vi "AB_Engine_Get_User_Build_Data.vi"(11 "Build in":refnum<class "AB_Build.lvclass">) -> (0 "Build Spec Name":string, 1 "Project Path":path, 2 "Main Destination":path, 3 "Build out":refnum<class "AB_Build.lvclass">, 4 "Target Name":string, 6 "Always Included VIs":path[](array[path]))   [LabVIEW 2020]
uses:
  <vilib>/AppBuilder/AB_Classes/Build/AB_Build.lvclass
  <vilib>/AppBuilder/AB_Classes/Source/AB_Source.lvclass
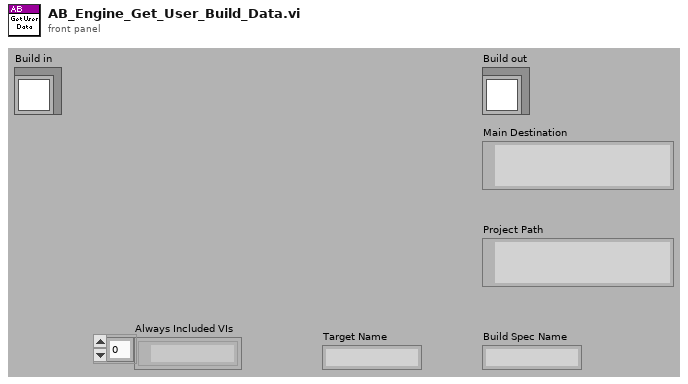
[diagram p1: front panel]
types:
  T1 = typedef "AB_Build.ctl" = cluster{"buildSpecName":string, "buildSpecDescription":string, "destinations":refnum<class "AB_Destination.lvclass">[], "exclusionOption":T2, "defaultLanguage":string, "supportedLanguages":string[], "excludedDirectories":path[], "buildContext":refnum<vi>, "buildObject":T3, "preview":bool, "programatic":bool, "progressBarEvents":T4, "userLog_Path":path, "preActionID":string, "preAction_Path":path, "postActionID":string, "postAction_Path":path, "eng_checkForBrokenVIs?":bool, "eng_verboseLinkerErrors?":bool, "localDest_Path":path, "targetDest_Path":path, "removeVIObject":u16, "cache":refnum<class "PreviewCache.lvclass">, "use cache":bool, "previewCache_ID":string, "buildCache_ID":string, "eng_TempLocalDest_Path":path, "eng_collectDependencies?":bool, "versionInfo":cluster{"buildVersion":cluster{"major":u16, "minor":u16, "patch":u16, "build":u16}, "autoIncrement":bool}, "eng_enableVIChecksums":bool}
  T2 = typedef "AB_Exclusion_Option.ctl" = cluster{"typedefs":bool, "polymorphicVIs":bool, "unusedLibraryItems":bool, "modifyLibraryFile":bool, "edit-timeDependencies":bool, "inlineVIs":bool, "dependent PPLs":bool, "dependent DLLs":bool}
  T3 = typedef "ItemRef.ctl" = u64
  T4 = typedef "provcom_ProgressBar_Events.ctl" = cluster{"newJob":refnum<user-event>, "newItem":refnum<user-event>, "errorMsg":T5, "cancel":refnum<user-event>}
  T5 = typedef "mxLvBuildError.ctl" = refnum<user-event>
  T6 = cluster{"major":u16, "minor":u16, "patch":u16, "build":u16}
  T7 = typedef "AB_Source.ctl" = cluster{"path":path, "itemID":string, "parentIndex":i32, "sourceInclusion":T8, "destinationIndex":i32, "properties":T9[], "newName":string, "lvfile":bool, "valid":bool, "eng_inBuild":bool, "eng_isNonVILink":bool, "Amalgamation":bool, "Amalgamation Piece":bool, "eng_delimitedName":string, "preventRename":bool}
  T8 = typedef "AB_Source_Inclusion.ctl" = enum16{"IncludeIfReferenced", "Include", "Exclude", "TopLevel"}
  T9 = typedef "AB_Source_Properties.ctl" = cluster{"sourcePropertyType":T10, "value":variant}
  T10 = typedef "AB_Source_Property_Type.ctl" = enum16{"Remove block diagram", "Remove front panel", "Password", "Window has title bar", "Show menu bar", "Show vertical scroll bar", "Show horizontal scroll bar", "Show toolbar", "Show Abort button", "Show fp when called", "Window behavior", "Allow user to close window", "Window run-time position", "Run when opened", "Allow debugging", "Auto error handling", "Generate guard code", "Use stack variables", "Expression folding", "Integer only", "Inline subVI"}
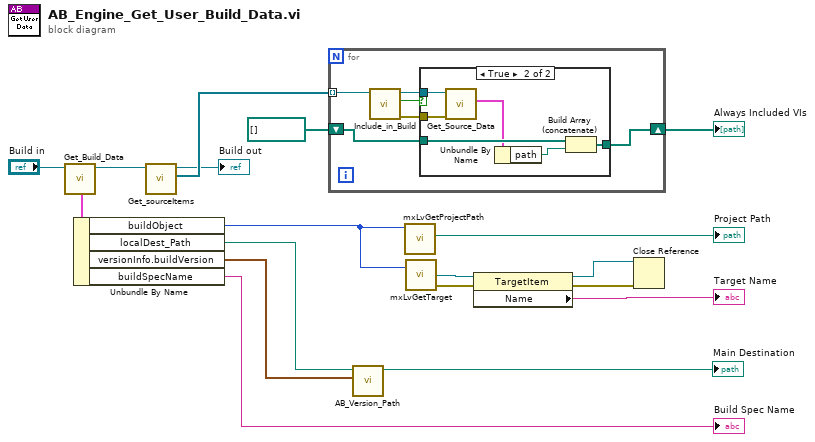
[diagram p0: block diagram]
diagram:
  n1 = call <vilib>:"Get_Build_Data.vi"("Class in"="Build in") -> ("data"=w7:T1, "Class out"=w5:refnum<class "AB_Build.lvclass">)  [unwired: 1 in, 8 out]
  n2 = Unbundle By Name(w7) -> ("buildObject"=w13:T3, "localDest_Path"=w2:path, "versionInfo.buildVersion"=w3:T6, "buildSpecName"=→"Build Spec Name":string)
  n3 = call <vilib>:"Get_sourceItems.vi"("Class in"=w5) -> ("sourceItems"=w6:refnum<class "AB_Source.lvclass">[], "Class out"=→"Build out":refnum<class "AB_Build.lvclass">)  [unwired: 8 in, 1 out]
  n4 = for {
    shift-right: [w21] -> w18
    shift-left: path[] [] ("appended array") -> [w22]
    tunnel: w6 -> [w19] mode=indexing
    n5 = call-dynamic "Include_in_Build.vi"("AB_Source in"=w19) -> ("error out"=w20:errorcluster, "includeInBuild"=w23:bool, "AB_Source out"=w24:refnum<class "AB_Source.lvclass">)  [unwired: 8 in]
    n6 = case shown="True" w23 {
      tunnel: w24 -> [_ w31]
      tunnel: w22 -> [w25 w30]
      tunnel: [w25 w29] -> w21
      tunnel: w20 -> [_ w28]
      frame False {
      }
      frame True {
        n7 = call <vilib>:"Get_Source_Data.vi"("error in (no error)"=w28, "Class in"=w31) -> ("data"=w27:T7)  [unwired: 7 in, 2 out]
        n8 = Unbundle By Name(w27) -> ("path"=w26:path)
        n9 = Build Array (concatenate)(w30, w26) -> (w29:path[])
      }
    }
  }
  "Always Included VIs" <- w18
  n10 = call <vilib>:"AB_Version_Path.vi"("buildVersion"=w3, "unversioned path"=w2) -> ("versioned path"=→"Main Destination":path)  [unwired: 9 in]
  n11 = call <resource>:"mxLvGetProjectPath.vi"("Item"=w13) -> ("Project Path"=→"Project Path":path)  [unwired: 8 in, 2 out]
  n12 = call <resource>:"mxLvGetTarget.vi"("Item"=w13) -> ("Target"=w15:refnum<vi>, "error out"=w14:errorcluster)  [unwired: 1 in, 1 out]
  n13 = property class="TargetItem"(reference=w15, error in=w14) -> (reference out=w10:refnum<vi>, error out=w9:errorcluster, "Name"=→"Target Name":string)
  n14 = Close Reference(reference=w10, error in (no error)=w9) -> ()  [unwired: 1 out]
